vi "KISSIA_TO ARRAY_MIDE_FLUJOS.vi"(10 "String":string="Mide Bronkhorst 1, mide Alicats 0,  y pausa 1.0s") -> (1 "Array":string[](array[string]))   [LabVIEW 2017]
panel:
  # "Mide Bronkhorst 1, mide Alicats 0,  y pausa 1.0s"
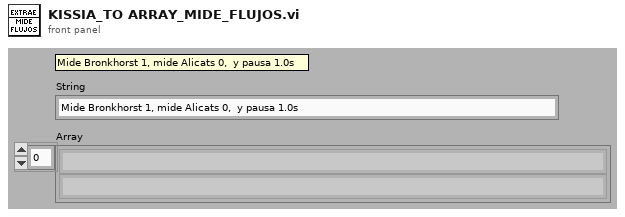
[diagram p1: front panel]
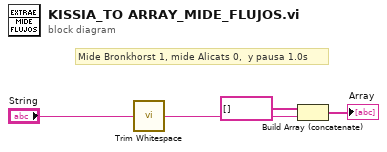
[diagram p0: block diagram]
diagram:
  # "Mide Bronkhorst 1, mide Alicats 0,  y pausa 1.0s"
  n1 = call <vilib>:"Trim Whitespace.vi"("string"="String") -> ("trimmed string"=w1:string)  [unwired: 1 in]
  n2 = Build Array (concatenate)(string[] [] ("Array I"), w1) -> (→"Array":string[])
